vi "extract_and_process_image.vi"(0 "Image Q In":T3, 2 "Threshold range":cluster{"Lower value":sgl, "Upper value":sgl}={"Lower value"=6.0, "Upper value"=1024.0}, 7 "Processed Image Data In":T2) -> (4 "error out":errorcluster, 8 "Processed Image Data Out":T2, 13 "Count data":T1)   [LabVIEW 2023]
uses:
  <vilib>/vision/Image Controls.llb/IMAQ Image.ctl
panel:
  in  "Number of Images":u32=10000000
  out "Image Q Out":T3
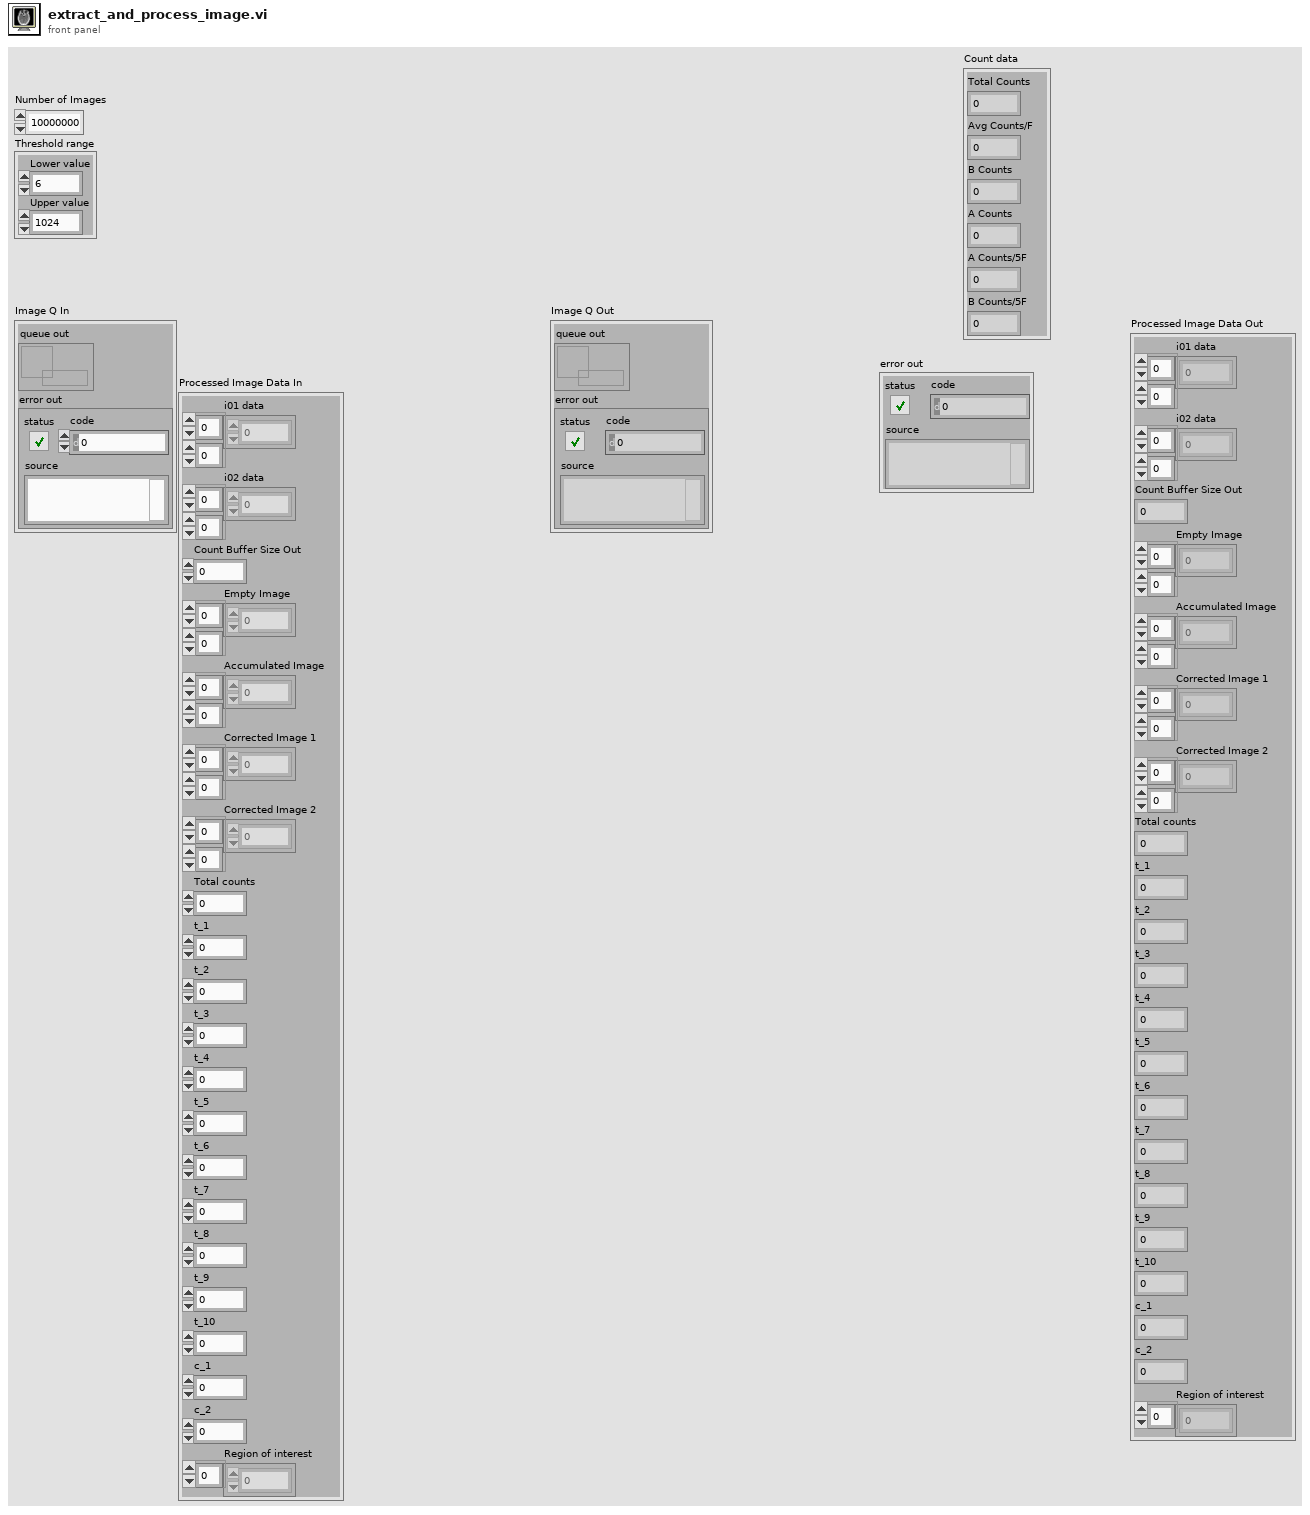
[diagram p1: front panel]
types:
  T1 = cluster{"Total Counts":u32, "Avg Counts/F":dbl, "B Counts":u32, "A Counts":u32, "A Counts/5F":dbl, "B Counts/5F":dbl}
  T2 = cluster{"i01 data":sgl[][], "i02 data":sgl[][], "Count Buffer Size Out":i32, "Empty Image":i16[][], "Accumulated Image":i16[][], "Corrected Image 1":i16[][], "Corrected Image 2":i16[][], "Total counts":i32, "t_1":i32, "t_2":i32, "t_3":i32, "t_4":i32, "t_5":i32, "t_6":i32, "t_7":i32, "t_8":i32, "t_9":i32, "t_10":i32, "c_1":i32, "c_2":i32, "Region of interest":i32[]}
  T3 = cluster{"queue out":refnum<queue>, "error out":errorcluster}
  T4 = typedef "IMAQ Image.ctl" = refnum<image>
  T5 = cluster{"Image Out":T4, "Image Data":cluster{"Actual Width":u32, "Actual Height":u32, "Buffer Number":i32}, "Imaging Variables In":cluster{"Region of interest":i32[], "Number of buffers":u32, "Frame timeout (ms)":u32}}
  T6 = cluster{"Accumulated Image":i16[][], "Particle Measurements (Pixels)":dbl[][], "Number of Particles":u16}
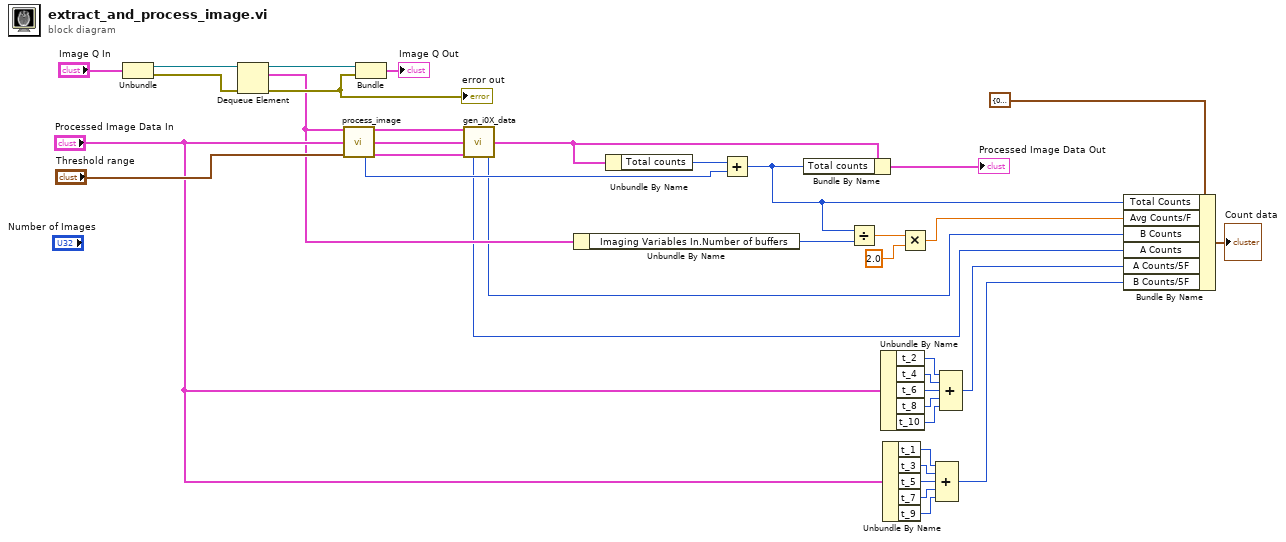
[diagram p0: block diagram]
diagram:
  n1 = Unbundle("Image Q In") -> ("queue out"=w35:refnum<queue>, "error out"=w34:errorcluster)
  n2 = Dequeue Element(queue=w35, error in (no error)=w34) -> (queue out=w33:refnum<queue>, element=w11:T5, error out=w32:errorcluster)  [unwired: 1 in, 1 out]
  "error out" <- w32
  n3 = call "process_image.vi"("Image Data In"=w11, "Image Processing Data In"="Processed Image Data In", "Threshold range"="Threshold range") -> ("Image Data Out"=w29:T5, "Image Processing Data Out"=w28:T2, "Number of Particles"=w15:u16, "Output data"=w27:T6)  [unwired: 7 in, 2 out]
  n4 = Bundle("queue out"=w33, "error out"=w32) -> (→"Image Q Out":T3)  [unwired: 1 in]
  n5 = call "gen_i0X_data.vi"("Raw Image Data In"=w29, "Processed Image Data In"=w28, "Input data"=w27) -> ("Processed Image Data In Out"=w14:T2, "A Counts"=w4:u32, "B Counts"=w5:u32)  [unwired: 9 in, 1 out]
  n6 = Unbundle By Name(w11) -> ("Imaging Variables In.Number of buffers"=w10:u32)
  n7 = Unbundle By Name(w14) -> ("Total counts"=w16:i32)
  n8 = Add(x=w16, y=w15) -> (x+y=w7:i32)
  n9 = Bundle By Name(cluster=w14, "Total counts"=w7) -> (→"Processed Image Data Out":T2)
  n10 = Divide(x=w7, y=w10) -> (x/y=w12:dbl)
  n11 = Unbundle By Name("Processed Image Data In") -> ("t_2"=w26:i32, "t_4"=w25:i32, "t_6"=w24:i32, "t_8"=w23:i32, "t_10"=w22:i32)
  n12 = Unbundle By Name("Processed Image Data In") -> ("t_1"=w21:i32, "t_3"=w20:i32, "t_5"=w2:i32, "t_7"=w19:i32, "t_9"=w18:i32)
  n13 = Multiply(x=w12, y=2.0) -> (x*y=w6:dbl)
  n14 = Compound Arithmetic op=ADD(w21, w20, w2, w19, w18) -> ()  [unwired: 1 out]
  n15 = Compound Arithmetic op=ADD(w26, w25, w24, w23, w22) -> (w3:i32)
  n16 = Bundle By Name(cluster=T1 {"Total Counts"=0, "Avg Counts/F"=0.0, "B Counts"=0, "A Counts"=0, "A Counts/5F"=0.0, "B Counts/5F"=0.0}, "Total Counts"=w7, "Avg Counts/F"=w6, "B Counts"=w5, "A Counts"=w4, "A Counts/5F"=w3, "B Counts/5F"=w2) -> (→"Count data":T1)
